vi "EEG_2022_040_LabView_5.3.vi"() -> ()   [LabVIEW 2022 SP3]
uses:
  Weather Data.ctl
panel:
  in  "Weather Data In":T1
  out "Weather Data Out":T1
  out "Error out":errorcluster
  in  "Error In":errorcluster
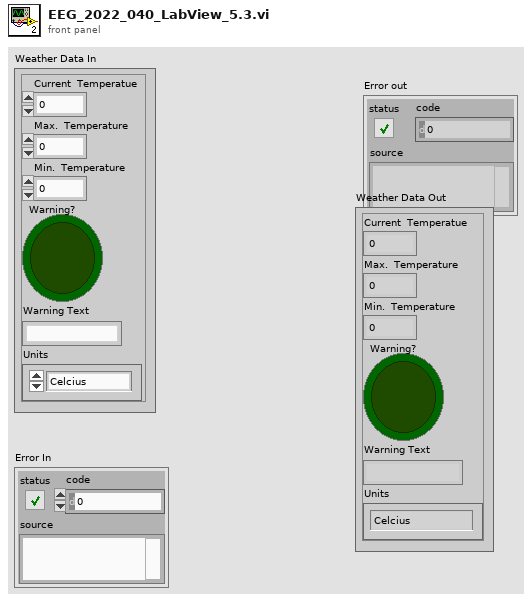
[diagram p1: front panel]
types:
  T1 = typedef "Weather Data.ctl" = cluster{"Current  Temperatue":dbl, "Max.  Temperature":dbl, "Min.  Temperature":dbl, "Warning?":bool, "Warning Text":string, "Units":enum16{"Celcius", "Fahrenheit"}}
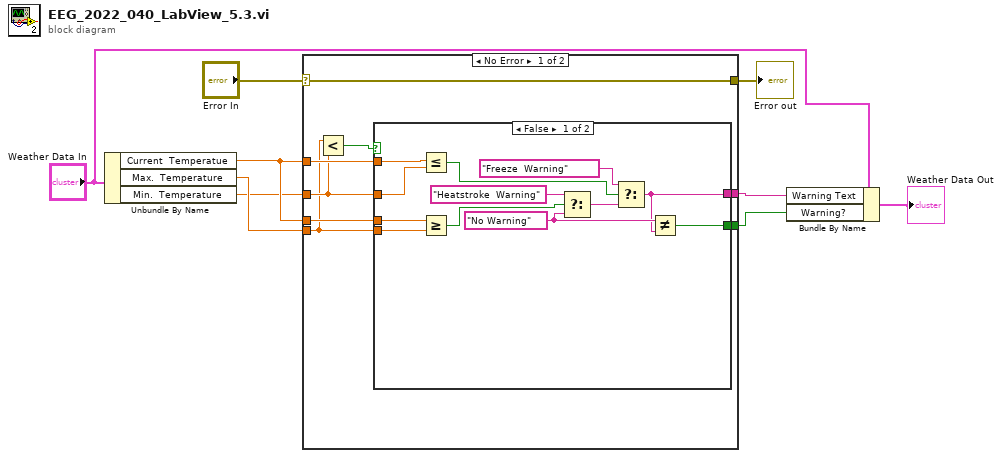
[diagram p0: block diagram]
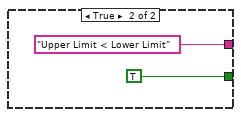
[diagram p2: hidden frame]
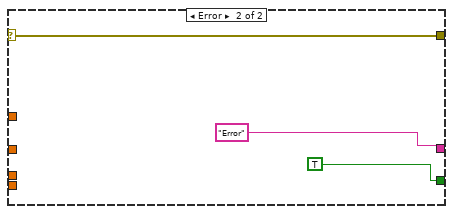
[diagram p3: hidden frame]
diagram:
  n1 = Unbundle By Name("Weather Data In") -> ("Current  Temperatue"=w6:dbl, "Max.  Temperature"=w7:dbl, "Min.  Temperature"=w5:dbl)
  n2 = case shown="No Error" "Error In" {
    selector: "Error In" -> [w17 w32]
    tunnel: [w17 w32] -> w9
    tunnel: [w15 "Error"] -> w3
    tunnel: [w14 TRUE] -> w4
    tunnel: w6 -> [w13 _]
    tunnel: w7 -> [w10 _]
    tunnel: w6 -> [w12 _]
    tunnel: w5 -> [w11 _]
    frame No Error {
      n3 = Less?(x=w10, y=w11) -> (x < y?=w16:bool)
      n4 = case shown="False" w16 {
        tunnel: [w23 "Upper Limit < Lower Limit"] -> w15
        tunnel: [w22 TRUE] -> w14
        tunnel: w13 -> [w21 _]
        tunnel: w10 -> [w20 _]
        tunnel: w12 -> [w19 _]
        tunnel: w11 -> [w18 _]
        frame False {
          w26 = "No Warning"
          n5 = Less Or Equal?(x=w19, y=w18) -> (x <= y?=w28:bool)
          n6 = Greater Or Equal?(x=w21, y=w20) -> (x >= y?=w27:bool)
          n7 = Select(t="Heatstroke  Warning", s=w27, f=w26) -> (s? t:f=w29:string)
          n8 = Select(t="Freeze  Warning", s=w28, f=w29) -> (s? t:f=w23:string)
          n9 = Not Equal?(x=w26, y=w23) -> (x != y?=w22:bool)
        }
        frame True {
        }
      }
    }
    frame Error {
    }
  }
  "Error out" <- w9
  n10 = Bundle By Name(cluster="Weather Data In", "Warning Text"=w3, "Warning?"=w4) -> (→"Weather Data Out":T1)
